vi "PH_Sound.Haenschen 2.vi"() -> (0 "... ist auch wohlgemut.":cluster{"Tone":dbl, "Beats":i32}[](array[cluster]))   [LabVIEW 2009, in "PH_Sound.lvlib"]
doc: "\"... ist auch wohlgemut.\""
uses:
  PH_Sound.lvlib
  PH_Common/PH_Audio/PH_3Oktaves.ctl
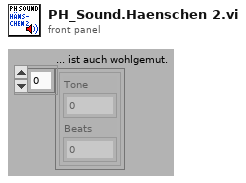
[diagram p1: front panel]
types:
  T1 = typedef "PH_3Oktaves.ctl" = dbl
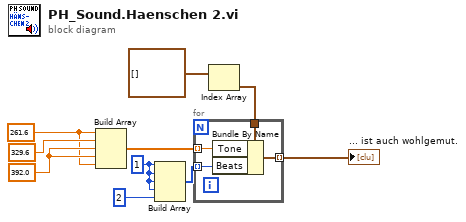
[diagram p0: block diagram]
diagram:
  w6 = T1 392.0 items=["c"=130.8, "cis"=138.6, "d"=146.8, "es"=155.6, "e"=164.8, "f"=174.6, "fis"=185.0, "g"=196.0, "as"=207.6, "a"=220.0, "b"=233.1, "h"=246.9, "c'"=261.6, "cis'"=277.2, "d'"=293.7, "es'"=311.1, "e'"=329.6, "f'"=349.2, "fis'"=370.0, "g'"=392.0, "as'"=415.3, "a'"=440.0, "b'"=466.2, "h'"=493.9, "c''"=523.3, "cis''"=554.4, "d''"=587.3, "es''"=622.3, "e''"=659.3, "f''"=689.5, "fis''"=740.0, "g''"=784.0, "as''"=830.6, "a''"=880.0, "b''"=932.3, "h''"=987.8, "c'''"=1047.0] ("3 Octaves")
  w7 = T1 329.6 items=["c"=130.8, "cis"=138.6, "d"=146.8, "es"=155.6, "e"=164.8, "f"=174.6, "fis"=185.0, "g"=196.0, "as"=207.6, "a"=220.0, "b"=233.1, "h"=246.9, "c'"=261.6, "cis'"=277.2, "d'"=293.7, "es'"=311.1, "e'"=329.6, "f'"=349.2, "fis'"=370.0, "g'"=392.0, "as'"=415.3, "a'"=440.0, "b'"=466.2, "h'"=493.9, "c''"=523.3, "cis''"=554.4, "d''"=587.3, "es''"=622.3, "e''"=659.3, "f''"=689.5, "fis''"=740.0, "g''"=784.0, "as''"=830.6, "a''"=880.0, "b''"=932.3, "h''"=987.8, "c'''"=1047.0] ("3 Octaves")
  w5 = T1 261.6 items=["c"=130.8, "cis"=138.6, "d"=146.8, "es"=155.6, "e"=164.8, "f"=174.6, "fis"=185.0, "g"=196.0, "as"=207.6, "a"=220.0, "b"=233.1, "h"=246.9, "c'"=261.6, "cis'"=277.2, "d'"=293.7, "es'"=311.1, "e'"=329.6, "f'"=349.2, "fis'"=370.0, "g'"=392.0, "as'"=415.3, "a'"=440.0, "b'"=466.2, "h'"=493.9, "c''"=523.3, "cis''"=554.4, "d''"=587.3, "es''"=622.3, "e''"=659.3, "f''"=689.5, "fis''"=740.0, "g''"=784.0, "as''"=830.6, "a''"=880.0, "b''"=932.3, "h''"=987.8, "c'''"=1047.0] ("3 Octaves")
  w1 = u32 1 ("element")
  n1 = Build Array(w5, w7, w6, w6, w5) -> (w4:T1[])
  n2 = Build Array(w1, w1, w1, w1, u32 2 ("y")) -> (w3:u32[])
  n3 = Index Array(array=cluster{"Tone":dbl, "Beats":i32}[] [] ("Song")) -> (element=w8:cluster{"Tone":dbl, "Beats":i32})  [unwired: 1 in]
  n4 = for {
    tunnel: w4 -> [w13] mode=indexing
    tunnel: w3 -> [w12] mode=indexing
    tunnel: w8 -> [w14]
    tunnel: [w11] -> w10 mode=indexing
    n5 = Bundle By Name(cluster=w14, "Tone"=w13, "Beats"=w12) -> (w11:cluster{"Tone":dbl, "Beats":i32})
  }
  "... ist auch wohlgemut." <- w10
